vi "Analog Tasks.vi"() -> ()   [LabVIEW 2017]
panel:
  out "physical channels 2":string="DemoDevice,BID#0/ai0:1" caption="property value"
  out "physical channels 1":string="DemoDevice,BID#0/ai0:1" caption="property value"
  out "property value":string="USB-4704,BID#0/ai0:7"
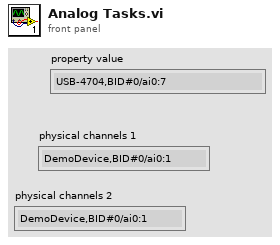
[diagram p1: front panel]
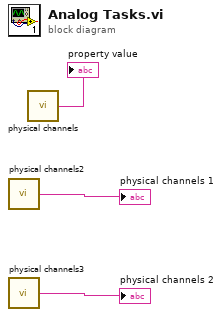
[diagram p0: block diagram]
diagram:
  n1 = call "physical channels2"() -> ("property value"=→"physical channels 1":string)  [unwired: 1 out]
  n2 = call "physical channels3"() -> ("property value"=→"physical channels 2":string)  [unwired: 1 out]
  n3 = call "physical channels"() -> ("property value"=→"property value":string)  [unwired: 1 out]
